vi "Parser_0x52_(SubVI).vi"(8 "error in":errorcluster, 9 "float":bool=TRUE, 11 "String in":string) -> (0 "error out":errorcluster, 1 "кол-во считанных байт тела запрошенного параметра":i32, 2 "Начальное смещение в байтах":i32, 3 "Номер табличного параметра":i32, 4 "ArrayFract32":fxp<+/-,32,1>[](array[numeric]), 6 "ArrayFloat":sgl[](array[numeric]))   [LabVIEW 2017, in "LV_Unicorn.lvlib"]
uses:
  LV_Unicorn.lvlib
panel:
  out "length 2":i32
  out "Size":i32
  out "String in 2":string
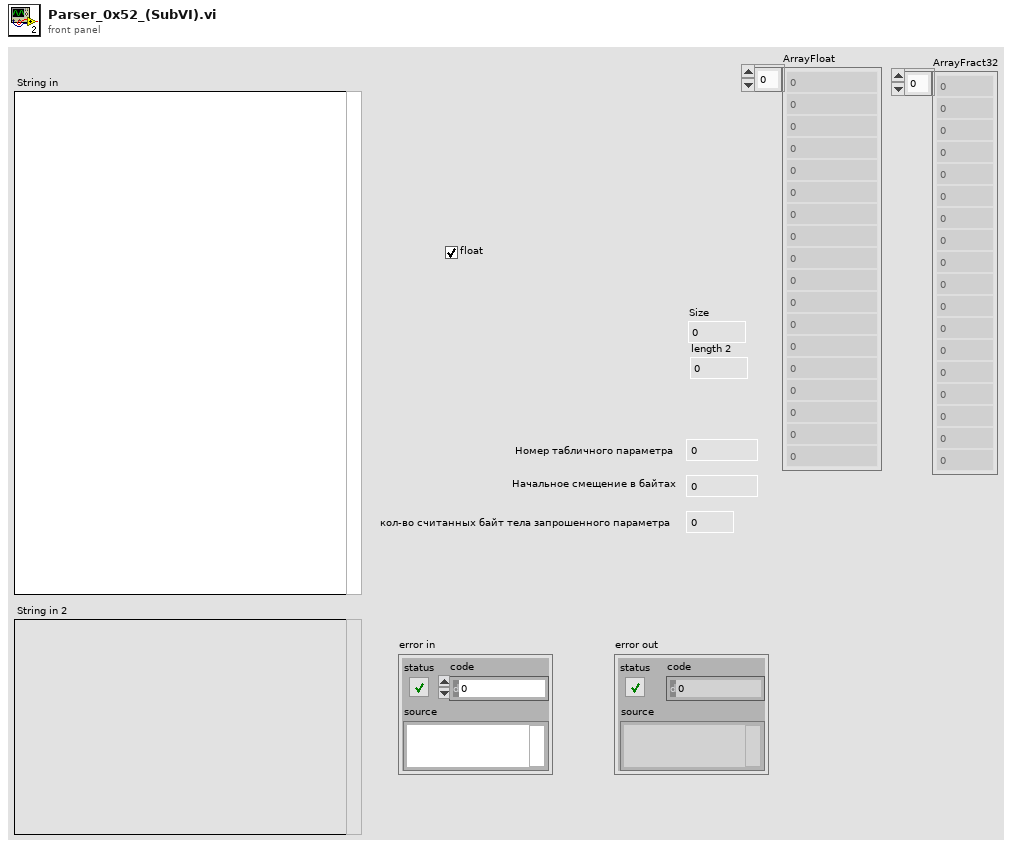
[diagram p1: front panel]
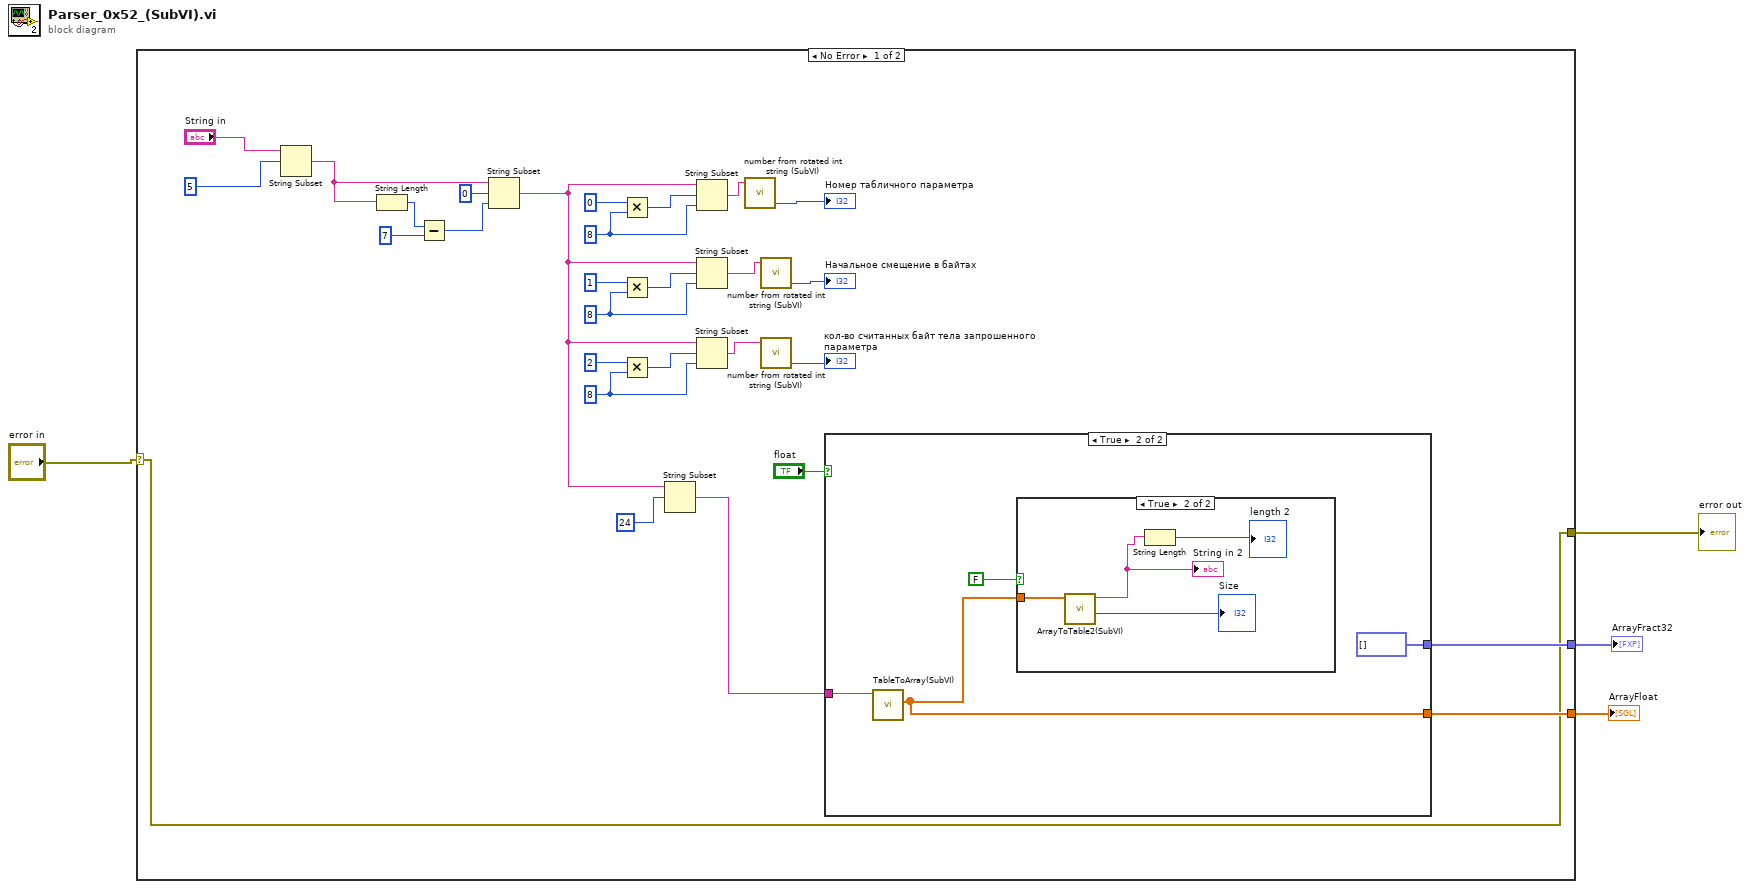
[diagram p0: block diagram]
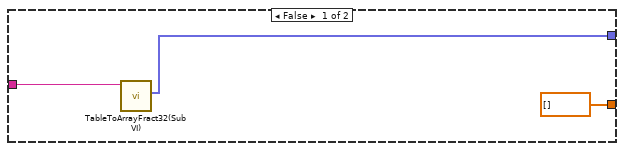
[diagram p2: hidden frame]
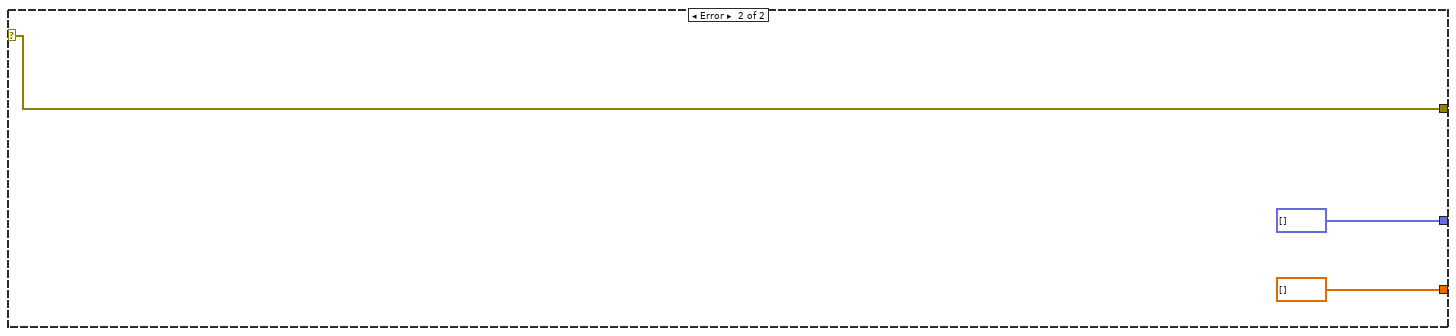
[diagram p4: hidden frame]
diagram:
  n1 = case shown="No Error" "error in" {
    selector: "error in" -> [w5 w45]
    tunnel: [w7 sgl[] [] ("Array")] -> w3
    tunnel: [w6 fxp<+/-,32,1>[] [] ("Array")] -> w2
    tunnel: [w5 w45] -> w1
    frame No Error {
      w13 = u32 8 ("length (rest)")
      w16 = u32 8 ("length (rest)")
      w21 = u32 8 ("length (rest)")
      n2 = String Subset(string="String in", offset (0)=5) -> (substring=w23:string)  [unwired: 1 in]
      n3 = String Length(string=w23) -> (length=w28:i32)
      n4 = Subtract(x=w28, y=7) -> (x-y=w24:i32)
      n5 = String Subset(string=w23, offset (0)=0, length (rest)=w24) -> (substring=w11:string)
      n6 = Multiply(x=u32 0, y=w13) -> (x*y=w14:u32)
      n7 = Multiply(x=u32 1, y=w16) -> (x*y=w15:u32)
      n8 = Multiply(x=u32 2, y=w21) -> (x*y=w22:u32)
      n9 = String Subset(string=w11, offset (0)=24) -> (substring=w25:string)  [unwired: 1 in]
      n10 = String Subset(string=w11, offset (0)=w14, length (rest)=w13) -> (substring=w9:string)
      n11 = String Subset(string=w11, offset (0)=w15, length (rest)=w16) -> (substring=w10:string)
      n12 = String Subset(string=w11, offset (0)=w22, length (rest)=w21) -> (substring=w19:string)
      n13 = call "number from rotated int string (SubVI).vi"("String"=w9) -> ("int number"=→"Номер табличного параметра":i32)  [unwired: 2 in, 2 out]
      n14 = call "number from rotated int string (SubVI).vi"("String"=w10) -> ("int number"=→"Начальное смещение в байтах":i32)  [unwired: 2 in, 2 out]
      n15 = call "number from rotated int string (SubVI).vi"("String"=w19) -> ("int number"=→"кол-во считанных байт тела запрошенного параметра":i32)  [unwired: 2 in, 2 out]
      n16 = case shown="True" "float" {
        tunnel: w25 -> [w36 w40]
        tunnel: [sgl[] [] ("Array") w38] -> w7
        tunnel: [w35 fxp<+/-,32,1>[] [] ("Array")] -> w6
        frame False {
          n17 = call "TableToArrayFract32(SubVI).vi"("String in"=w36) -> ("Array"=w35:fxp<+/-,32,1>[])  [unwired: 10 in]
        }
        frame True {
          n18 = call "TableToArray(SubVI).vi"("String in"=w40) -> ("Array"=w38:sgl[])  [unwired: 10 in]
          n19 = case shown="True" FALSE {
            tunnel: w38 -> [_ w44]
            frame False {
            }
            frame True {
              n20 = call "ArrayToTable2(SubVI).vi"("Table1D"=w44) -> ("Size"=→"Size":i32, "String"=w42:string)  [unwired: 9 in]
              "String in 2" <- w42
              n21 = String Length(string=w42) -> (length=→"length 2":i32)
            }
          }
        }
      }
    }
    frame Error {
    }
  }
  "error out" <- w1
  "ArrayFloat" <- w3
  "ArrayFract32" <- w2
